vi "Clean up.vi"(8 "error in (no error)":errorcluster, 11 "Analyze Compound Analysis Base in":refnum<class "Analyze Compound Analysis Base.lvclass">) -> (0 "error out":errorcluster, 3 "Analyze Compound Analysis Base out":refnum<class "Analyze Compound Analysis Base.lvclass">)   [LabVIEW 2020, in "Analyze.lvlib" / "Analyze Compound Analysis Base.lvclass"]
uses:
  Analyze Compound Analysis Base.lvclass
  Analyze BaseClass/Analyze BaseClass/Analyze BaseClass.lvclass
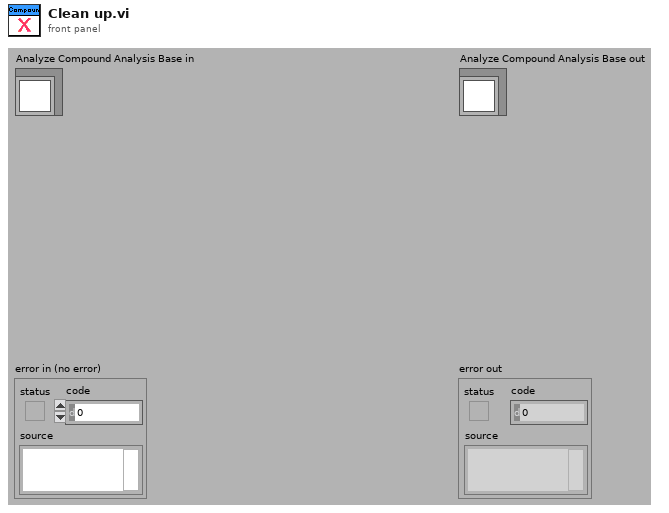
[diagram p1: front panel]
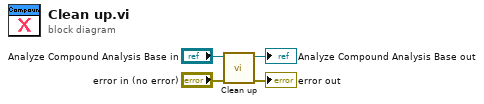
[diagram p0: block diagram]
diagram:
  n1 = call-parent "Clean up.vi"("error in (no error)"="error in (no error)", "Analyze BaseClass in"="Analyze Compound Analysis Base in") -> ("error out"=→"error out":errorcluster, "Analyze BaseClass out"=→"Analyze Compound Analysis Base out":refnum<class "Analyze Compound Analysis Base.lvclass">)  [unwired: 8 in]
